vi "灭火装置监测界面.vi"() -> ()   [LabVIEW 2016, in "环境动力监测库.lvlib"]
panel:
  out "烟雾告警":bool
  out "温度":sgl(knob) scale=0.0..100.0
  in  "解除告警":bool
  out "x+1":u32
  out "灭火装置监测":bool caption="状态"
  out "告警内容":string
  out "灭火装置信号持续时间":u32=60 format="%.0fS"
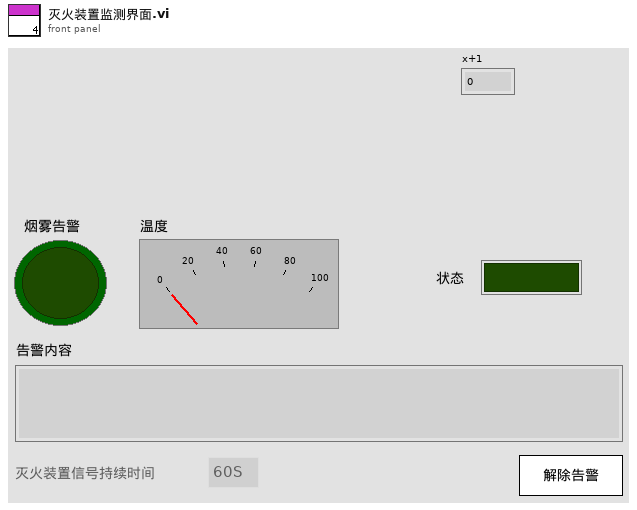
[diagram p1: front panel]
types:
  T1 = cluster{"漏水监测输出":cluster{"漏水监测告警":bool, "告警内容":string}, "门禁监测输出":cluster{"门禁监测告警":bool, "告警内容":string}, "门禁监测输出2":cluster{"门禁监测告警":bool, "告警内容":string}, "温湿度监测输出":cluster{"温湿度监测告警":bool, "告警内容":string}, "烟雾监测输出":cluster{"烟雾监测告警":bool, "告警内容":string}, "空调监测输出":cluster{"空调监测告警":bool, "告警内容":string}, "自动重合闸输出":cluster{"自动重合闸告警":bool, "告警内容":string}, "红外入侵输出":cluster{"红外入侵告警":bool, "告警内容":string}, "振动输出":cluster{"振动告警":bool, "告警内容":string}, "UPS输出":cluster{"UPS告警":bool, "告警内容":string}, "蓄电池输出":cluster{"蓄电池告警":bool, "告警内容":string}, "蓄电池输出2":cluster{"蓄电池告警":bool, "告警内容":string}, "GPS输出":cluster{"定位告警":bool, "告警内容":string}, "北斗输出":cluster{"定位告警":bool, "告警内容":string}, "气象输出":cluster{"气象告警":bool, "告警内容":string}, "废液输出":cluster{"废液告警":bool, "告警内容":string}, "废液输出2":cluster{"废液告警":bool, "告警内容":string}, "灭火装置输出":cluster{"灭火装置告警":bool, "告警内容":string}}
  T2 = cluster{"温湿度":cluster{"状态":bool, "温度:":sgl, "湿度:":sgl, "详情  ":bool}, "空调":cluster{"状态":bool, "机柜温度:":sgl, "压缩机:":enum16{"停止", "运行"}, "电加热:":enum16{"停止", "运行"}, "详情  ":bool}, "排气扇":cluster{"排气扇":bool, "详情  ":bool}, "冰箱":cluster{"冰箱":bool, "详情  ":bool}}
  T3 = cluster{"漏水监测配置":cluster{"监测项描述:输出":string, "端口":enum16{"AI0", "AI1", "AI2", "AI3", "AI4", "DI0", "DI1", "DI2", "DI3", "DI4", "DI5", "DI6", "DI7", "DO0", "DO1", "DO2", "DO3", "DO4", "DO5", "DO6", "DO7", "X0", "X1", "X2", "X3", "X4", "X5", "X6", "X7", "X8", "X9", "X10", "X11", "X12", "X13", "X14", "X15", "X16", "X17", "X18", "X19", "X20", "X21", "X22", "X23", "Y0", "Y1", "Y2", "Y3", "Y4", "Y5", "Y6", "Y7", "Y8", "Y9", "Y10", "Y11", "Y12", "Y13", "Y14", "Y15", "Y16", "Y17", "Y18", "Y19", "Y20", "Y21", "Y22", "Y23", "Y24", "Y25", "Y26", "Y27", "Y28", "Y29", "Y30", "Y31", "Y32", "Y33", "Y34", "Y35", "Y36", "Y37", "Y38", "Y39"}, "告警参数:":enum32{"禁用告警", "闭合告警", "断开告警"}, "传感器型号:":enum16{"PLC", "ZLAN", "ART"}, "声光告警启用":bool}, "门禁开关监测配置":cluster{"监测项描述:输出":string, "端口":enum16{"AI0", "AI1", "AI2", "AI3", "AI4", "DI0", "DI1", "DI2", "DI3", "DI4", "DI5", "DI6", "DI7", "DO0", "DO1", "DO2", "DO3", "DO4", "DO5", "DO6", "DO7", "X0", "X1", "X2", "X3", "X4", "X5", "X6", "X7", "X8", "X9", "X10", "X11", "X12", "X13", "X14", "X15", "X16", "X17", "X18", "X19", "X20", "X21", "X22", "X23", "Y0", "Y1", "Y2", "Y3", "Y4", "Y5", "Y6", "Y7", "Y8", "Y9", "Y10", "Y11", "Y12", "Y13", "Y14", "Y15", "Y16", "Y17", "Y18", "Y19", "Y20", "Y21", "Y22", "Y23", "Y24", "Y25", "Y26", "Y27", "Y28", "Y29", "Y30", "Y31", "Y32", "Y33", "Y34", "Y35", "Y36", "Y37", "Y38", "Y39"}, "告警参数:":enum32{"禁用告警", "闭合告警", "断开告警"}, "传感器型号:":enum16{"PLC", "ZLAN", "ART"}, "声光告警启用":bool}, "门禁开关监测配置2":cluster{"监测项描述:输出":string, "端口":enum16{"AI0", "AI1", "AI2", "AI3", "AI4", "DI0", "DI1", "DI2", "DI3", "DI4", "DI5", "DI6", "DI7", "DO0", "DO1", "DO2", "DO3", "DO4", "DO5", "DO6", "DO7", "X0", "X1", "X2", "X3", "X4", "X5", "X6", "X7", "X8", "X9", "X10", "X11", "X12", "X13", "X14", "X15", "X16", "X17", "X18", "X19", "X20", "X21", "X22", "X23", "Y0", "Y1", "Y2", "Y3", "Y4", "Y5", "Y6", "Y7", "Y8", "Y9", "Y10", "Y11", "Y12", "Y13", "Y14", "Y15", "Y16", "Y17", "Y18", "Y19", "Y20", "Y21", "Y22", "Y23", "Y24", "Y25", "Y26", "Y27", "Y28", "Y29", "Y30", "Y31", "Y32", "Y33", "Y34", "Y35", "Y36", "Y37", "Y38", "Y39"}, "告警参数:":enum32{"禁用告警", "闭合告警", "断开告警"}, "传感器型号:":enum16{"PLC", "ZLAN", "ART"}, "声光告警启用":bool}, "温湿度监测配置":cluster{"监测项描述:输出":string, "端口":enum16{"AI0", "AI1", "AI2", "AI3", "AI4", "DI0", "DI1", "DI2", "DI3", "DI4", "DI5", "DI6", "DI7", "DO0", "DO1", "DO2", "DO3", "DO4", "DO5", "DO6", "DO7", "X0", "X1", "X2", "X3", "X4", "X5", "X6", "X7", "X8", "X9", "X10", "X11", "X12", "X13", "X14", "X15", "X16", "X17", "X18", "X19", "X20", "X21", "X22", "X23", "Y0", "Y1", "Y2", "Y3", "Y4", "Y5", "Y6", "Y7", "Y8", "Y9", "Y10", "Y11", "Y12", "Y13", "Y14", "Y15", "Y16", "Y17", "Y18", "Y19", "Y20", "Y21", "Y22", "Y23", "Y24", "Y25", "Y26", "Y27", "Y28", "Y29", "Y30", "Y31", "Y32", "Y33", "Y34", "Y35", "Y36", "Y37", "Y38", "Y39"}, "告警参数:":enum32{"禁用告警", "闭合告警", "断开告警"}, "传感器型号:":enum16{"PLC", "ZLAN", "ART"}, "声光告警启用":bool}, "烟雾监测配置":cluster{"监测项描述:输出":string, "端口":enum16{"AI0", "AI1", "AI2", "AI3", "AI4", "DI0", "DI1", "DI2", "DI3", "DI4", "DI5", "DI6", "DI7", "DO0", "DO1", "DO2", "DO3", "DO4", "DO5", "DO6", "DO7", "X0", "X1", "X2", "X3", "X4", "X5", "X6", "X7", "X8", "X9", "X10", "X11", "X12", "X13", "X14", "X15", "X16", "X17", "X18", "X19", "X20", "X21", "X22", "X23", "Y0", "Y1", "Y2", "Y3", "Y4", "Y5", "Y6", "Y7", "Y8", "Y9", "Y10", "Y11", "Y12", "Y13", "Y14", "Y15", "Y16", "Y17", "Y18", "Y19", "Y20", "Y21", "Y22", "Y23", "Y24", "Y25", "Y26", "Y27", "Y28", "Y29", "Y30", "Y31", "Y32", "Y33", "Y34", "Y35", "Y36", "Y37", "Y38", "Y39"}, "告警参数:":enum32{"禁用告警", "闭合告警", "断开告警"}, "传感器型号:":enum16{"PLC", "ZLAN", "ART"}, "声光告警启用":bool}, "冰箱监测配置":cluster{"监测项描述:输出":string, "端口":enum16{"AI0", "AI1", "AI2", "AI3", "AI4", "DI0", "DI1", "DI2", "DI3", "DI4", "DI5", "DI6", "DI7", "DO0", "DO1", "DO2", "DO3", "DO4", "DO5", "DO6", "DO7", "X0", "X1", "X2", "X3", "X4", "X5", "X6", "X7", "X8", "X9", "X10", "X11", "X12", "X13", "X14", "X15", "X16", "X17", "X18", "X19", "X20", "X21", "X22", "X23", "Y0", "Y1", "Y2", "Y3", "Y4", "Y5", "Y6", "Y7", "Y8", "Y9", "Y10", "Y11", "Y12", "Y13", "Y14", "Y15", "Y16", "Y17", "Y18", "Y19", "Y20", "Y21", "Y22", "Y23", "Y24", "Y25", "Y26", "Y27", "Y28", "Y29", "Y30", "Y31", "Y32", "Y33", "Y34", "Y35", "Y36", "Y37", "Y38", "Y39"}, "告警参数:":enum32{"禁用告警", "闭合告警", "断开告警"}, "传感器型号:":enum16{"PLC", "ZLAN", "ART"}, "声光告警启用":bool}, "排气扇监测配置":cluster{"监测项描述:输出":string, "端口":enum16{"AI0", "AI1", "AI2", "AI3", "AI4", "DI0", "DI1", "DI2", "DI3", "DI4", "DI5", "DI6", "DI7", "DO0", "DO1", "DO2", "DO3", "DO4", "DO5", "DO6", "DO7", "X0", "X1", "X2", "X3", "X4", "X5", "X6", "X7", "X8", "X9", "X10", "X11", "X12", "X13", "X14", "X15", "X16", "X17", "X18", "X19", "X20", "X21", "X22", "X23", "Y0", "Y1", "Y2", "Y3", "Y4", "Y5", "Y6", "Y7", "Y8", "Y9", "Y10", "Y11", "Y12", "Y13", "Y14", "Y15", "Y16", "Y17", "Y18", "Y19", "Y20", "Y21", "Y22", "Y23", "Y24", "Y25", "Y26", "Y27", "Y28", "Y29", "Y30", "Y31", "Y32", "Y33", "Y34", "Y35", "Y36", "Y37", "Y38", "Y39"}, "告警参数:":enum32{"禁用告警", "闭合告警", "断开告警"}, "传感器型号:":enum16{"PLC", "ZLAN", "ART"}, "声光告警启用":bool}, "红外入侵监测配置":cluster{"监测项描述:输出":string, "端口":enum16{"AI0", "AI1", "AI2", "AI3", "AI4", "DI0", "DI1", "DI2", "DI3", "DI4", "DI5", "DI6", "DI7", "DO0", "DO1", "DO2", "DO3", "DO4", "DO5", "DO6", "DO7", "X0", "X1", "X2", "X3", "X4", "X5", "X6", "X7", "X8", "X9", "X10", "X11", "X12", "X13", "X14", "X15", "X16", "X17", "X18", "X19", "X20", "X21", "X22", "X23", "Y0", "Y1", "Y2", "Y3", "Y4", "Y5", "Y6", "Y7", "Y8", "Y9", "Y10", "Y11", "Y12", "Y13", "Y14", "Y15", "Y16", "Y17", "Y18", "Y19", "Y20", "Y21", "Y22", "Y23", "Y24", "Y25", "Y26", "Y27", "Y28", "Y29", "Y30", "Y31", "Y32", "Y33", "Y34", "Y35", "Y36", "Y37", "Y38", "Y39"}, "告警参数:":enum32{"禁用告警", "闭合告警", "断开告警"}, "传感器型号:":enum16{"PLC", "ZLAN", "ART"}, "声光告警启用":bool}, "振动监测配置":cluster{"监测项描述:输出":string, "端口":enum16{"AI0", "AI1", "AI2", "AI3", "AI4", "DI0", "DI1", "DI2", "DI3", "DI4", "DI5", "DI6", "DI7", "DO0", "DO1", "DO2", "DO3", "DO4", "DO5", "DO6", "DO7", "X0", "X1", "X2", "X3", "X4", "X5", "X6", "X7", "X8", "X9", "X10", "X11", "X12", "X13", "X14", "X15", "X16", "X17", "X18", "X19", "X20", "X21", "X22", "X23", "Y0", "Y1", "Y2", "Y3", "Y4", "Y5", "Y6", "Y7", "Y8", "Y9", "Y10", "Y11", "Y12", "Y13", "Y14", "Y15", "Y16", "Y17", "Y18", "Y19", "Y20", "Y21", "Y22", "Y23", "Y24", "Y25", "Y26", "Y27", "Y28", "Y29", "Y30", "Y31", "Y32", "Y33", "Y34", "Y35", "Y36", "Y37", "Y38", "Y39"}, "告警参数:":enum32{"禁用告警", "闭合告警", "断开告警"}, "传感器型号:":enum16{"PLC", "ZLAN", "ART"}, "声光告警启用":bool}, "废液监测配置":cluster{"监测项描述:输出":string, "端口":enum16{"AI0", "AI1", "AI2", "AI3", "AI4", "DI0", "DI1", "DI2", "DI3", "DI4", "DI5", "DI6", "DI7", "DO0", "DO1", "DO2", "DO3", "DO4", "DO5", "DO6", "DO7", "X0", "X1", "X2", "X3", "X4", "X5", "X6", "X7", "X8", "X9", "X10", "X11", "X12", "X13", "X14", "X15", "X16", "X17", "X18", "X19", "X20", "X21", "X22", "X23", "Y0", "Y1", "Y2", "Y3", "Y4", "Y5", "Y6", "Y7", "Y8", "Y9", "Y10", "Y11", "Y12", "Y13", "Y14", "Y15", "Y16", "Y17", "Y18", "Y19", "Y20", "Y21", "Y22", "Y23", "Y24", "Y25", "Y26", "Y27", "Y28", "Y29", "Y30", "Y31", "Y32", "Y33", "Y34", "Y35", "Y36", "Y37", "Y38", "Y39"}, "告警参数:":enum32{"禁用告警", "闭合告警", "断开告警"}, "传感器型号:":enum16{"PLC", "ZLAN", "ART"}, "声光告警启用":bool}, "废液监测配置2":cluster{"监测项描述:输出":string, "端口":enum16{"AI0", "AI1", "AI2", "AI3", "AI4", "DI0", "DI1", "DI2", "DI3", "DI4", "DI5", "DI6", "DI7", "DO0", "DO1", "DO2", "DO3", "DO4", "DO5", "DO6", "DO7", "X0", "X1", "X2", "X3", "X4", "X5", "X6", "X7", "X8", "X9", "X10", "X11", "X12", "X13", "X14", "X15", "X16", "X17", "X18", "X19", "X20", "X21", "X22", "X23", "Y0", "Y1", "Y2", "Y3", "Y4", "Y5", "Y6", "Y7", "Y8", "Y9", "Y10", "Y11", "Y12", "Y13", "Y14", "Y15", "Y16", "Y17", "Y18", "Y19", "Y20", "Y21", "Y22", "Y23", "Y24", "Y25", "Y26", "Y27", "Y28", "Y29", "Y30", "Y31", "Y32", "Y33", "Y34", "Y35", "Y36", "Y37", "Y38", "Y39"}, "告警参数:":enum32{"禁用告警", "闭合告警", "断开告警"}, "传感器型号:":enum16{"PLC", "ZLAN", "ART"}, "声光告警启用":bool}, "灭火装置监测配置":cluster{"监测项描述:输出":string, "端口":enum16{"AI0", "AI1", "AI2", "AI3", "AI4", "DI0", "DI1", "DI2", "DI3", "DI4", "DI5", "DI6", "DI7", "DO0", "DO1", "DO2", "DO3", "DO4", "DO5", "DO6", "DO7", "X0", "X1", "X2", "X3", "X4", "X5", "X6", "X7", "X8", "X9", "X10", "X11", "X12", "X13", "X14", "X15", "X16", "X17", "X18", "X19", "X20", "X21", "X22", "X23", "Y0", "Y1", "Y2", "Y3", "Y4", "Y5", "Y6", "Y7", "Y8", "Y9", "Y10", "Y11", "Y12", "Y13", "Y14", "Y15", "Y16", "Y17", "Y18", "Y19", "Y20", "Y21", "Y22", "Y23", "Y24", "Y25", "Y26", "Y27", "Y28", "Y29", "Y30", "Y31", "Y32", "Y33", "Y34", "Y35", "Y36", "Y37", "Y38", "Y39"}, "告警参数:":enum32{"禁用告警", "闭合告警", "断开告警"}, "传感器型号:":enum16{"PLC", "ZLAN", "ART"}, "声光告警启用":bool}}
  T4 = cluster{"监测项描述:输出":string, "端口":enum16{"AI0", "AI1", "AI2", "AI3", "AI4", "DI0", "DI1", "DI2", "DI3", "DI4", "DI5", "DI6", "DI7", "DO0", "DO1", "DO2", "DO3", "DO4", "DO5", "DO6", "DO7", "X0", "X1", "X2", "X3", "X4", "X5", "X6", "X7", "X8", "X9", "X10", "X11", "X12", "X13", "X14", "X15", "X16", "X17", "X18", "X19", "X20", "X21", "X22", "X23", "Y0", "Y1", "Y2", "Y3", "Y4", "Y5", "Y6", "Y7", "Y8", "Y9", "Y10", "Y11", "Y12", "Y13", "Y14", "Y15", "Y16", "Y17", "Y18", "Y19", "Y20", "Y21", "Y22", "Y23", "Y24", "Y25", "Y26", "Y27", "Y28", "Y29", "Y30", "Y31", "Y32", "Y33", "Y34", "Y35", "Y36", "Y37", "Y38", "Y39"}, "告警参数:":enum32{"禁用告警", "闭合告警", "断开告警"}, "传感器型号:":enum16{"PLC", "ZLAN", "ART"}, "声光告警启用":bool}
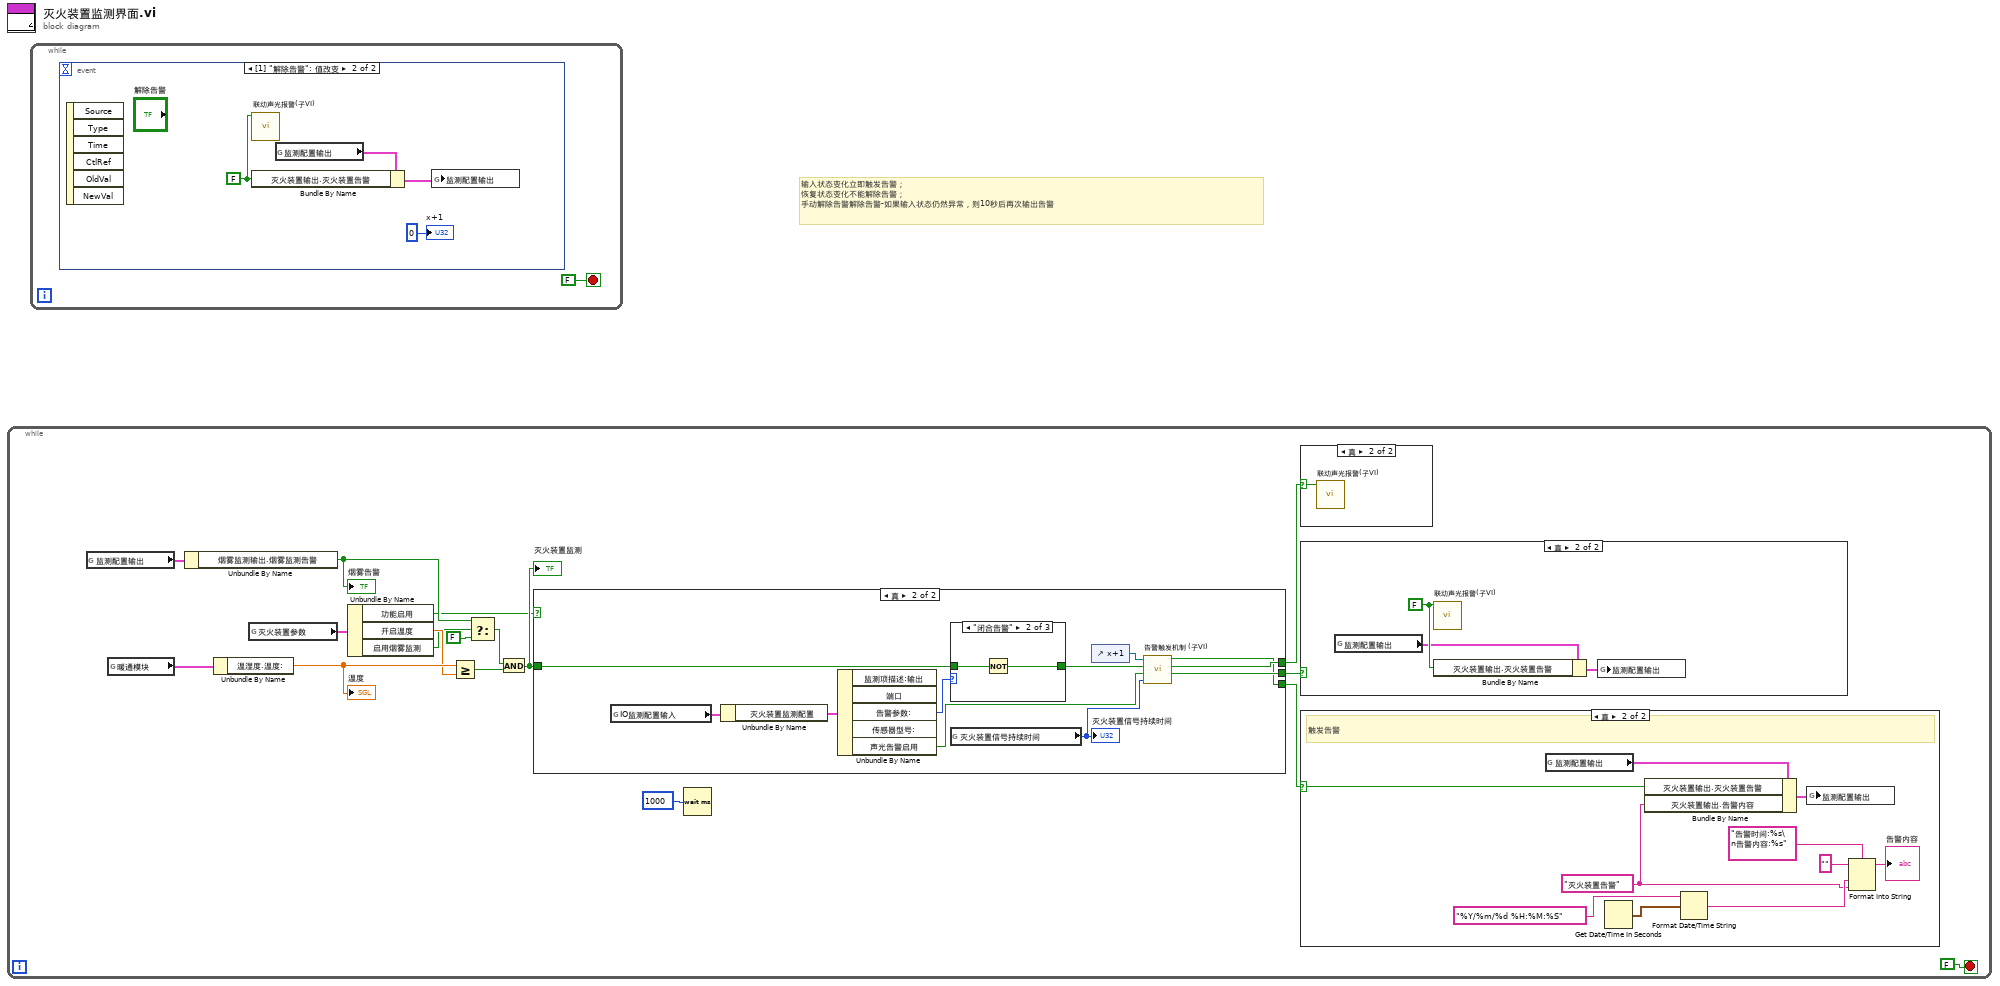
[diagram p0: block diagram]
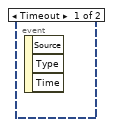
[diagram p2: hidden frame]
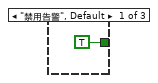
[diagram p4: hidden frame]
diagram:
  # "输入状态变化立即触发告警；\n恢复状态变化不能解除告警；\n手动解除告警解除告警-如果输入状态仍然异常，则10秒后再次输出告警"
  n1 = while {
    stop <- FALSE stop-if-true
    n2 = global read "内部交互全局变量.vi" "监测配置输出"() -> (w13:T1)
    n3 = global read "内部交互全局变量.vi" "暖通模块"() -> (w12:T2)
    n4 = Unbundle By Name(w13) -> ("烟雾监测输出.烟雾监测告警"=w5:bool)
    "烟雾告警" <- w5
    n5 = Unbundle By Name(w12) -> ("温湿度.温度:"=w10:sgl)
    "温度" <- w10
    n6 = global read "断电保存全局变量.vi" "灭火装置参数"() -> (w8:cluster{"功能启用":bool, "开启温度":dbl, "启用烟雾监测":bool})
    n7 = Unbundle By Name(w8) -> ("功能启用"=w1:bool, "开启温度"=w7:dbl, "启用烟雾监测"=w6:bool)
    n8 = Greater Or Equal?(x=w10, y=w7) -> (x >= y?=w11:bool)
    n9 = Select(t=w5, s=w6, f=FALSE) -> (s? t:f=w3:bool)
    n10 = And(x=w3, y=w11) -> (x .and. y?=w2:bool)
    "灭火装置监测" <- w2
    n11 = case shown="真" w1 {
      tunnel: [_ w28] -> w15
      tunnel: [_ w24] -> w14
      tunnel: [_ w19] -> w9
      tunnel: w2 -> [_ w18]
      frame False {
      }
      frame True {
        n12 = global read "断电保存全局变量.vi" "IO监测配置输入"() -> (w23:T3)
        n13 = Unbundle By Name(w23) -> ("灭火装置监测配置"=w22:T4)
        n14 = Unbundle By Name(w22) -> ("告警参数:"=w21:enum32{"禁用告警", "闭合告警", "断开告警"}, "声光告警启用"=w20:bool)  [unwired: 3 out]
        n15 = case shown="\"闭合告警\"" w21 {
          tunnel: w18 -> [_ w31 w32]
          tunnel: [TRUE ("漏水监测输出") w30 w32] -> w27
          frame "禁用告警", Default {
          }
          frame "闭合告警" {
            n16 = Not(x=w31) -> (.not. x?=w30:bool)
          }
          frame "断开告警" {
          }
        }
        n17 = global read "断电保存全局变量.vi" "灭火装置信号持续时间"() -> (w25:u32)
        "灭火装置信号持续时间" <- w25
        n18 = control-ref of="x+1"() -> (w26:refnum<vi>)
        n19 = call "告警触发机制 (子VI).vi"("信号持续时间"=w25, "声光告警启用"=w20, "状态输出真-正常"=w27, "Digital输入"=w26) -> ("消除告警"=w24:bool, "声光告警"=w28:bool, "触发告警"=w19:bool)  [unwired: 5 in]
      }
    }
    n20 = Wait (ms)(milliseconds to wait=u32 1000 ("等待时间（毫秒）")) -> ()  [unwired: 1 out]
    n21 = case shown="真" w15 {
      selector: w15 -> [_ w36]
      frame False {
      }
      frame True {
        n22 = call "联动声光报警(子VI).vi"("布尔"=w36) -> ()  [unwired: 11 in]
      }
    }
    n23 = case shown="真" w14 {
      frame False {
      }
      frame True {
        w35 = FALSE
        n24 = global read "内部交互全局变量.vi" "监测配置输出"() -> (w34:T1)
        n25 = call "联动声光报警(子VI).vi"("布尔"=w35) -> ()  [unwired: 11 in]
        n26 = Bundle By Name(cluster=w34, "灭火装置输出.灭火装置告警"=w35) -> (w33:T1)
        n27 = global write "内部交互全局变量.vi" "监测配置输出"(w33) -> ()
      }
    }
    n28 = case shown="真" w9 {
      selector: w9 -> [_ w46]
      frame False {
      }
      frame True {
        w37 = "灭火装置告警" ("报警内容")
        # "触发告警"
        n29 = global read "内部交互全局变量.vi" "监测配置输出"() -> (w38:T1)
        n30 = Get Date/Time In Seconds() -> (seconds since 1Jan1904=w43:timestamp)
        n31 = Bundle By Name(cluster=w38, "灭火装置输出.灭火装置告警"=w46, "灭火装置输出.告警内容"=w37) -> (w39:T1)
        n32 = Format Date/Time String(time format string (%c)="%Y/%m/%d %H:%M:%S" ("时间格式字符串(%c)"), seconds (now)=w43) -> (date/time string=w45:string)  [unwired: 1 in]
        n33 = global write "内部交互全局变量.vi" "监测配置输出"(w39) -> ()
        n34 = Format Into String(format string="告警时间:%s\n告警内容:%s" ("格式字符串"), initial string="" ("初始字符串"), w45, w37) -> (resulting string=→"告警内容":string)  [unwired: 1 in, 1 out]
      }
    }
  }
  n35 = while {
    stop <- FALSE stop-if-true
    n36 = event shown="[1] \"解除告警\": 值改变" {
      selector: _ -> [_ _]
      dyn-events: _ -> [_ _]
      timeout: _ -> [_ _]
      event Timeout {
        n37 = event-data() -> ()  [unwired: 1 in, 3 out]
      }
      event "解除告警": Value Change {
        w51 = FALSE
        n38 = event-data() -> ()  [unwired: 1 in, 6 out]
        n39 = call "联动声光报警(子VI).vi"("布尔"=w51) -> ()  [unwired: 11 in]
        n40 = global read "内部交互全局变量.vi" "监测配置输出"() -> (w49:T1)
        n41 = Bundle By Name(cluster=w49, "灭火装置输出.灭火装置告警"=w51) -> (w48:T1)
        n42 = global write "内部交互全局变量.vi" "监测配置输出"(w48) -> ()
        "x+1" <- u32 0 ("x+1")
      }
    }
  }
